vi "Constructor.vi"(8 "error in (no error)":errorcluster, 11 "ThinDough in":refnum<class "ThickDough.lvclass">) -> (0 "error out":errorcluster, 2 "Ingredients":string, 3 "ThinDough out":refnum<class "ThickDough.lvclass">)   [LabVIEW 2013, in "ThickDough.lvclass"]
uses:
  ThickDough.lvclass
panel:
  # "我是厚麵皮"
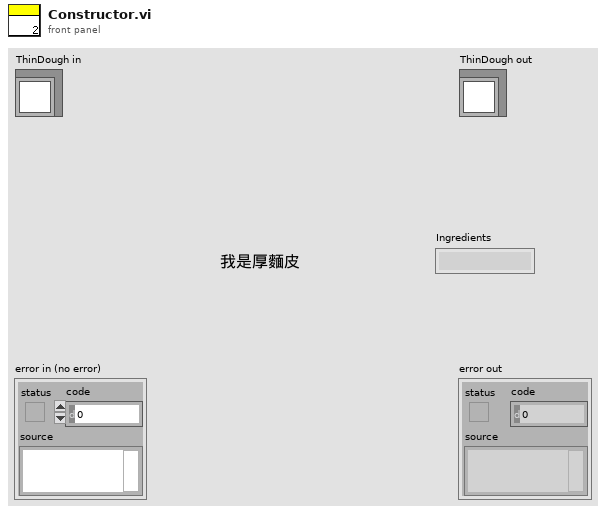
[diagram p1: front panel]
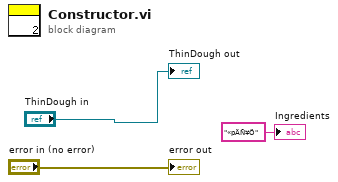
[diagram p0: block diagram]
diagram:
  "error out" <- "error in (no error)"
  "ThinDough out" <- "ThinDough in"
  "Ingredients" <- "«pÄÑ¥Ö" ("Ingredients")
